vi "ConfigInstr.vi"(6 "InstrumentName":string, 7 "VisaRessIn":refnum<visa-resource-name>, 8 "error in (no error)":errorcluster caption="entrée d'erreur (pas d'erreur)", 9 "FirstClassInst":bool, 10 "Function":string, 11 "GenData In":refnum<class "CoboltMLD.lvclass"> caption="DNL_LabVIEW Object in") -> (0 "error out":errorcluster caption="sortie d'erreur", 3 "GenData Out":refnum<class "CoboltMLD.lvclass"> caption="DNL_LabVIEW Object out")   [LabVIEW 2019, in "CoboltMLD.lvclass"]
uses:
  CoboltMLD.lvclass
  C:/Programmes Labview/LabScanV1A/DevicesClass/BaseDevice/BaseDevice.lvclass
  CoboltMLD_Func.ctl
  CoboltMLD.lvclass/CoboltMLD.ctl
  BaseDevice/BaseDevice.lvclass/BaseDevice.ctl
  BaseDevice/Accessor/SetShowInstrNm.vi
  BaseDevice/Accessor/SetInstrParam.vi
panel:
  in  "Class_Func":T1
  out "VisaRessOut":refnum<visa-resource-name>
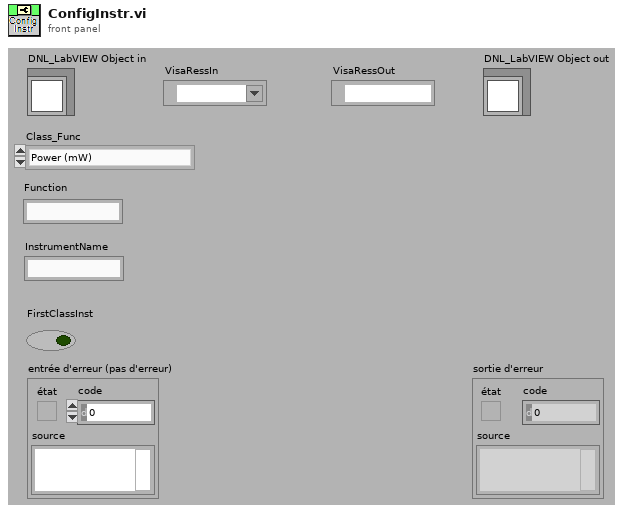
[diagram p1: front panel]
types:
  T1 = typedef "CoboltMLD.lvclass/CoboltMLD_Func.ctl" = enum16{"Power (mW)", "Current (mA)"}
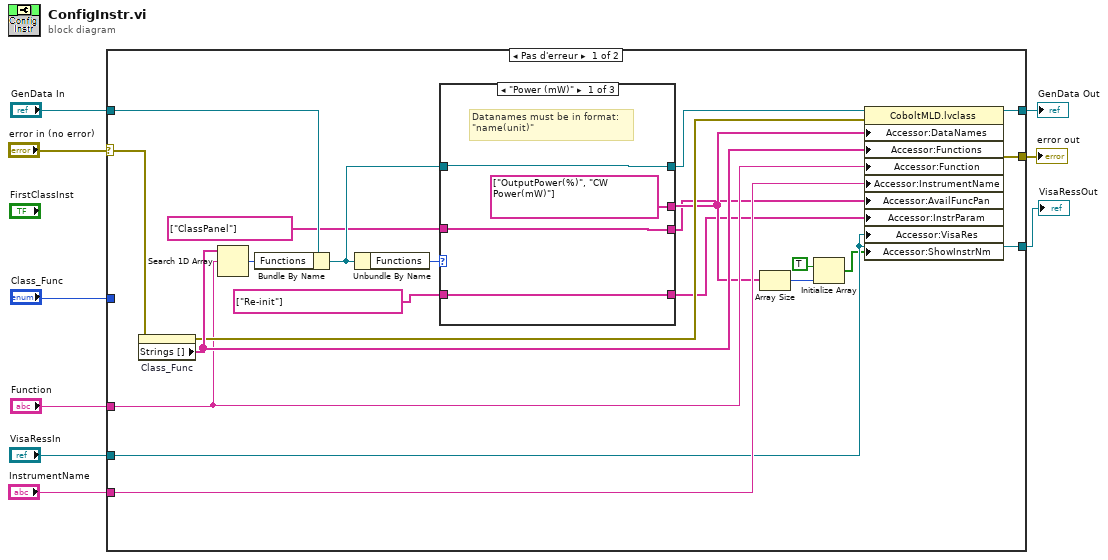
[diagram p0: block diagram]
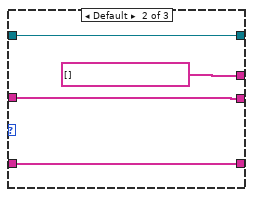
[diagram p2: hidden frame]
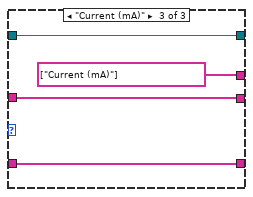
[diagram p3: hidden frame]
diagram:
  n1 = case shown="Pas d'erreur" "error in (no error)" {
    selector: "error in (no error)" -> [w24 w44]
    tunnel: [w30 w44] -> w8
    tunnel: "GenData In" -> [w25 w43]
    tunnel: [w29 w43] -> w6
    tunnel: "Class_Func" -> [_ _]
    tunnel: "Function" -> [w20 _]
    tunnel: "InstrumentName" -> [w19 _]
    tunnel: "VisaRessIn" -> [w18 _]
    tunnel: [w18 _] -> w1
    frame No Error {
      n2 = property on="Class_Func" class="Énum (strict)"(error in=w24) -> (error out=w23:errorcluster, "Strings []"=w27:string[])  [unwired: 1 in, 1 out]
      n3 = Search 1D Array(1D array=w27, element=w20) -> (index of element=w26:i32)  [unwired: 1 in]
      n4 = Bundle By Name(cluster=w25, "Functions"=w26) -> (w22:refnum<class "CoboltMLD.lvclass">)
      n5 = Unbundle By Name(w22) -> ("Functions"=w28:T1)
      n6 = case shown="\"Power (mW)\"" w28 {
        tunnel: [string[] ["OutputPower(%)", "CW Power(mW)"] string[] [] string[] ["Current (mA)"]] -> w15
        tunnel: w22 -> [w34 w38 w42]
        tunnel: [w34 w38 w42] -> w21
        tunnel: [w32 w36 w40] -> w11
        tunnel: [w31 w35 w39] -> w13
        tunnel: string[] ["ClassPanel"] -> [w32 w36 w40]
        tunnel: string[] ["Re-init"] -> [w31 w35 w39]
        frame "Power (mW)" {
          # "Datanames must be in format:\n\"name(unit)\""
        }
        frame Default {
        }
        frame "Current (mA)" {
        }
      }
      n7 = Array Size(array=w15) -> (size(s)=w17:i32)
      n8 = Initialize Array(TRUE, w17) -> (w14:bool[])
      n9 = property class="CoboltMLD.lvclass"(reference=w21, error in=w23, "Accessor:DataNames"=w15, "Accessor:Functions"=w27, "Accessor:Function"=w20, "Accessor:InstrumentName"=w19, "Accessor:AvailFuncPan"=w11, "Accessor:InstrParam"=w13, "Accessor:VisaRes"=w18, "Accessor:ShowInstrNm"=w14) -> (reference out=w29:refnum<class "CoboltMLD.lvclass">, error out=w30:errorcluster)
    }
    frame Error {
    }
  }
  "error out" <- w8
  "GenData Out" <- w6
  "VisaRessOut" <- w1
